vi "Basic Accuracy Parameter3.vi"(8 "error in (no error)":errorcluster, 11 "VISA resource name":refnum<visa-resource-name>) -> (0 "error out":errorcluster, 1 "Acal":dbl format="%.3f", 2 "Radcal":dbl format="%.3f", 3 "VISA resource name out":refnum<visa-resource-name>)   [LabVIEW 2015, in "Agilent 428X Series.lvlib"]
doc: "This control returns the value of calibration accuracy A Cal and Theta Cal.\n\nDisclaimer: All accuracy calculation VI's are not part of the original \n driver. They are provided for supplementry purpose only.\n If user desires very high accuracy data, please do or \n check the calculation seperately."
uses:
  <instrlib>/Agilent 428X Series/Agilent 428X Series.lvlib
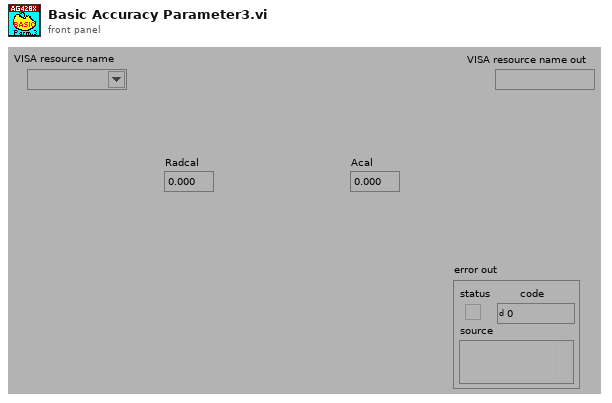
[diagram p1: front panel]
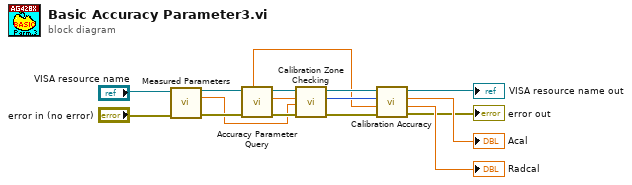
[diagram p0: block diagram]
diagram:
  n1 = call <instrlib>:"Measured Parameters.vi"("VISA resource name"="VISA resource name", "error in (no error)"="error in (no error)") -> ("VISA resource name out"=w5:refnum<visa-resource-name>, "Z"=w1:dbl, "error out"=w4:errorcluster)  [unwired: 7 in, 4 out]
  n2 = call <instrlib>:"Accuracy Parameter Query.vi"("error in (no error)"=w4, "VISA resource name"=w5) -> ("error out"=w12:errorcluster, "Voltage Level"=w16:dbl, "VISA resource name out"=w11:refnum<visa-resource-name>, "Frequency"=w6:dbl)  [unwired: 4 in, 2 out]
  n3 = call <instrlib>:"Calibration Zone Checking .vi"("error in (no error)"=w12, "Impedance Z (10m)"=w1, "Frequency (20)"=w16, "VISA resource name"=w11) -> ("error out"=w14:errorcluster, "Zone"=w13:i16, "VISA resource name out"=w15:refnum<visa-resource-name>)  [unwired: 5 in]
  n4 = call <instrlib>:"Calibration Accuracy.vi"("error in (no error)"=w14, "Frequency (20)"=w6, "Zone (0)"=w13, "VISA resource name"=w15) -> ("error out"=→"error out":errorcluster, "Radcal"=→"Radcal":dbl, "Acal"=→"Acal":dbl, "VISA resource name out"=→"VISA resource name out":refnum<visa-resource-name>)  [unwired: 4 in]
